vi "PNG tEXt Chunk.vi"(10 "Contents":string, 11 "Keyword":string) -> (3 "PNG Chunk":string)   [LabVIEW 2009]
doc: "Creates a PNG tEXt chunk.\n\nIn the format:\nKeyword /00 Data\n\nCode by Darin"
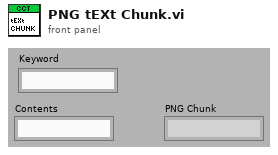
[diagram p1: front panel]
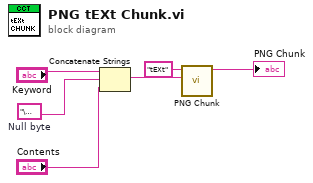
[diagram p0: block diagram]
diagram:
  w3 = "\u0000"  # Null byte
  n1 = Concatenate Strings("Keyword", w3, "Contents") -> (w1:string)
  n2 = call "PNG Chunk.vi"("Data"=w1, "Name"="tEXt") -> ("PNG Chunk"=→"PNG Chunk":string)  [unwired: 9 in]
